vi "FGV_MIDASSettingsFiles.vi"(6 "BinaryData":string, 7 "Enum":enum16{"AddData", "Set", "Get"}(ring), 8 "MD5 (optional)":string, 9 "FileName":string, 10 "ProjectName":string, 11 "Path":path) -> (1 "MD5 is same":bool, 2 "BinaryData":string, 3 "HaveData":bool)   [LabVIEW 2018, in "feGEM DataPacker.lvlib"]
uses:
  feGEM DataPacker.lvlib
  SettingsFileList.lvclass
  SettingsFileList.lvclass/SettingsFileList.ctl
  SettingsFile.lvclass/SettingsFile.ctl
  WriteDataToFile.vi
  GetBinaryData.vi
  CheckName.vi
  SetBinaryData.vi
  SettingsFile.lvclass
panel:
  out "SettingsFileList.lvclass 2":refnum<class "SettingsFileList.lvclass">
  in  "SettingsFileList.lvclass":refnum<class "SettingsFileList.lvclass">
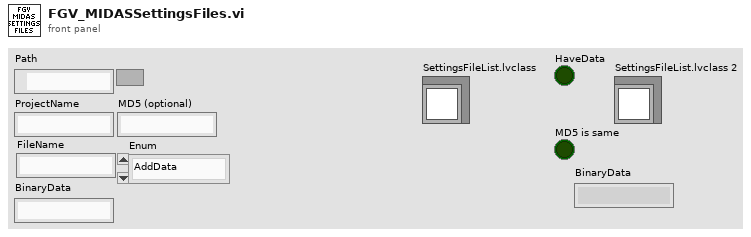
[diagram p1: front panel]
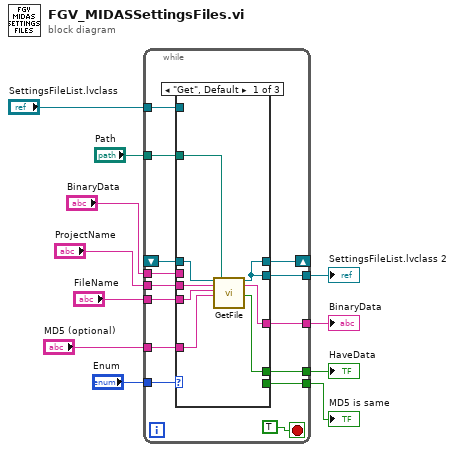
[diagram p0: block diagram]
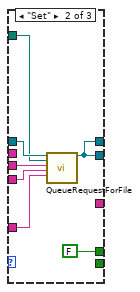
[diagram p2: hidden frame]
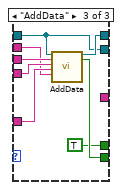
[diagram p3: hidden frame]
diagram:
  n1 = while {
    shift-right: [w24] -> _
    shift-left: _ -> [w25]
    tunnel: [w22] -> w10
    tunnel: "SettingsFileList.lvclass" -> [w21]
    tunnel: [w20] -> w9
    tunnel: "MD5 (optional)" -> [w19]
    tunnel: "FileName" -> [w18]
    tunnel: "ProjectName" -> [w17]
    tunnel: "Path" -> [w16]
    tunnel: "Enum" -> [w15]
    tunnel: [w14] -> w3
    tunnel: "BinaryData" -> [w13]
    tunnel: [w12] -> w1
    stop <- TRUE stop-if-true
    n2 = case shown="\"Get\", Default" w15 {
      tunnel: [w28 w35 w48] -> w24
      tunnel: w25 -> [w33 w40 w41]
      tunnel: [w28 w35 w41] -> w22
      tunnel: w21 -> [_ _ _]
      tunnel: [w27 _ _] -> w20
      tunnel: w19 -> [w30 w36 w44]
      tunnel: w18 -> [w31 w37 w45]
      tunnel: w17 -> [w32 w39 w46]
      tunnel: w16 -> [w29 w38 _]
      tunnel: [_ _ w47] -> w14
      tunnel: w13 -> [_ _ w43]
      tunnel: [w26 FALSE ("HaveData") TRUE ("HaveData")] -> w12
      frame "Get", Default {
        n3 = call "GetFile.vi"("SettingsFileList in"=w33, "ProjectName"=w32, "FileName"=w31, "MD5 (optional)"=w30, "Path"=w29) -> ("SettingsFileList out"=w28:refnum<class "SettingsFileList.lvclass">, "BinaryData"=w27:string, "HaveData"=w26:bool)  [unwired: 11 in, 1 out]
      }
      frame "Set" {
        n4 = call "QueueRequestForFile.vi"("SettingsFileList in"=w40, "Path"=w38, "ProjectName"=w39, "FileName"=w37, "MD5 (optional)"=w36) -> ("SettingsFileList out"=w35:refnum<class "SettingsFileList.lvclass">)  [unwired: 13 in, 1 out]
      }
      frame "AddData" {
        n5 = call "AddData.vi"("SettingsFileList in"=w41, "ProjectName"=w46, "FileName"=w45, "MD5 (optional)"=w44, "BinaryData"=w43) -> ("SettingsFileList out"=w48:refnum<class "SettingsFileList.lvclass">, "MD5 is same"=w47:bool)  [unwired: 12 in, 1 out]
      }
    }
  }
  "SettingsFileList.lvclass 2" <- w10
  "BinaryData" <- w9
  "MD5 is same" <- w3
  "HaveData" <- w1
